vi "splitEveData.vi"(9 "Clean Data Array":string[](array[string])) -> (0 "Energy":u32[](array[numeric]), 1 "Channel":u32[](array[numeric]), 2 "Chan+Energy":u32[](array[numeric]), 3 "Clk Ticks":u32[](array[numeric]), 4 "appended array":u32[][](array[numeric]), 5 "Sr No":u32[](array[numeric]))   [LabVIEW 2019]
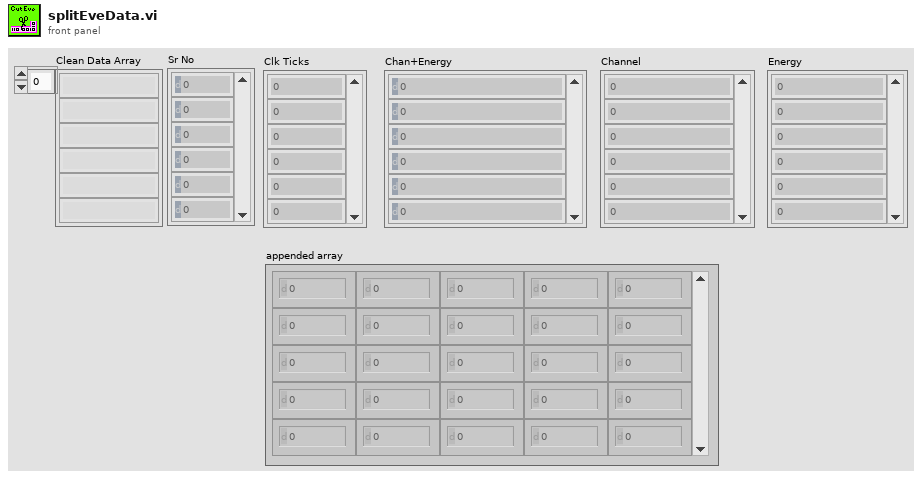
[diagram p1: front panel]
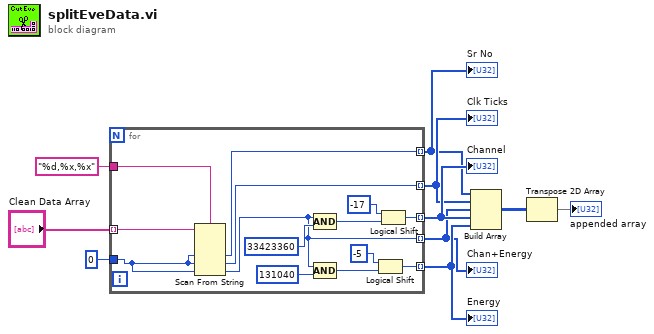
[diagram p0: block diagram]
diagram:
  n1 = for {
    tunnel: "Clean Data Array" -> [w24] mode=indexing
    tunnel: [w23] -> w1 mode=indexing
    tunnel: [w13] -> w2 mode=indexing
    tunnel: [w16] -> w3 mode=indexing
    tunnel: [w15] -> w7 mode=indexing
    tunnel: [w14] -> w4 mode=indexing
    tunnel: "%d,%x,%x" ("format string (%d,%x,%x)") -> [w12]
    tunnel: u32 0 -> [w11]
    n2 = Scan From String(format string=w12, input string=w24, default 1=w11, default 2=w11, default 3=w11) -> (output 1=w23:u32, output 2=w13:u32, output 3=w16:u32)  [unwired: 2 in, 3 out]
    n3 = Compound Arithmetic op=AND(w16, u32 33423360 ("value")) -> (w17:u32)
    n4 = Compound Arithmetic op=AND(w16, u32 131040 ("value")) -> (w20:u32)
    n5 = Logical Shift(y=-5, x=w20) -> (x << y=w14:u32)
    n6 = Logical Shift(y=-17, x=w17) -> (x << y=w15:u32)
  }
  "Sr No" <- w1
  "Clk Ticks" <- w2
  "Chan+Energy" <- w3
  "Energy" <- w4
  "Channel" <- w7
  n7 = Build Array(w1, w2, w3, w7, w4) -> (w5:u32[][])
  n8 = Transpose 2D Array(2D array=w5) -> (transposed array=→"appended array":u32[][])
